vi "ma_Spectrum Averaging (complex) no State.vi"(6 "state info":T2 {"real spectrum" format="%0.2f"; "averages completed" format="%0.2f"; "df" format="%0.2f"; "complex spectrum" format="%0.2f"; "spectrum parameters"."window" items=["Rectangle"=0, "Hanning"=1, "Hamming"=2, "Blackman-Harris"=3, "Exact Blackman"=4, "Blackman"=5, "Flat Top"=6, "4 Term B-Harris "=7, "7 Term B-Harris"=8, "Low Sidelobe"=9, "Blackman Nuttall"=11, "Triangle"=30, "Bartlett-Hanning"=31, "Bohman"=32, "Parzen"=33, "Welch"=34, "Kaiser"=60, "Dolph-Chebyshev"=61, "Gaussian"=62]; "dt" format="%0.2f"; "timestamp" format="%0.2f"; "dt history" format="%0.2f"; "t0 history" format="%0.2f"}, 7 "retrieve last spectrum (F)":bool, 8 "restart averaging (F)":bool, 9 "averaging parameters":T3={"averaging mode"=enum."No averaging", "weighting mode"=enum."Exponential", "number of averages"=10} {"number of averages" min=1}, 10 "df":dbl format="%0.2p", 11 "complex spectrum":cdb[](array[numeric]) format="%0.2p") -> (0 "averages completed":dbl format="%0.2f", 1 "averaging done":bool, 2 "df":dbl format="%0.2p", 3 "averaged complex spectrum":cdb[](array[numeric]) format="%0.2p", 4 "state info":T2 {"real spectrum" format="%0.2f"; "averages completed" format="%0.2f"; "df" format="%0.2f"; "complex spectrum" format="%0.2f"; "spectrum parameters"."window" items=["Rectangle"=0, "Hanning"=1, "Hamming"=2, "Blackman-Harris"=3, "Exact Blackman"=4, "Blackman"=5, "Flat Top"=6, "4 Term B-Harris "=7, "7 Term B-Harris"=8, "Low Sidelobe"=9, "Blackman Nuttall"=11, "Triangle"=30, "Bartlett-Hanning"=31, "Bohman"=32, "Parzen"=33, "Welch"=34, "Kaiser"=60, "Dolph-Chebyshev"=61, "Gaussian"=62]; "dt" format="%0.2f"; "timestamp" format="%0.2f"; "dt history" format="%0.2f"; "t0 history" format="%0.2f"})   [LabVIEW 2020, in "NI_MAPro.lvlib"]
uses:
  NI_MAPro.lvlib
  windowTd.ctl
  NI_AALPro.lvlib
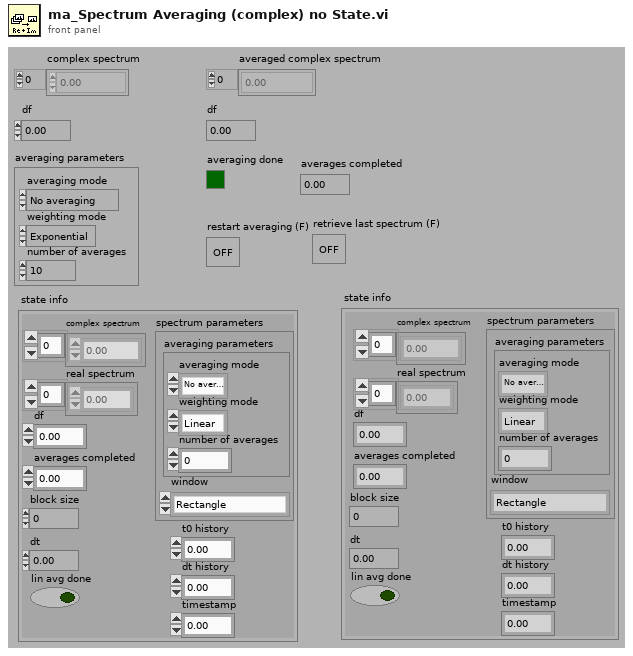
[diagram p1: front panel]
types:
  T1 = typedef "NI_AALPro.lvlib/windowTd.ctl" = u32
  T2 = cluster{"block size":i32, "dt":dbl, "spectrum parameters":cluster{"averaging parameters":cluster{"averaging mode":enum16{"No averaging", "Vector averaging", "RMS averaging", "Peak hold"}, "weighting mode":enum16{"Linear", "Exponential"}, "number of averages":u32}, "window":T1}, "df":dbl, "averages completed":dbl, "complex spectrum":cdb[], "real spectrum":dbl[], "t0 history":dbl, "dt history":dbl, "timestamp":dbl, "lin avg done":bool}
  T3 = cluster{"averaging mode":enum16{"No averaging", "Vector averaging", "RMS averaging", "Peak hold"}, "weighting mode":enum16{"Linear", "Exponential"}, "number of averages":u32}
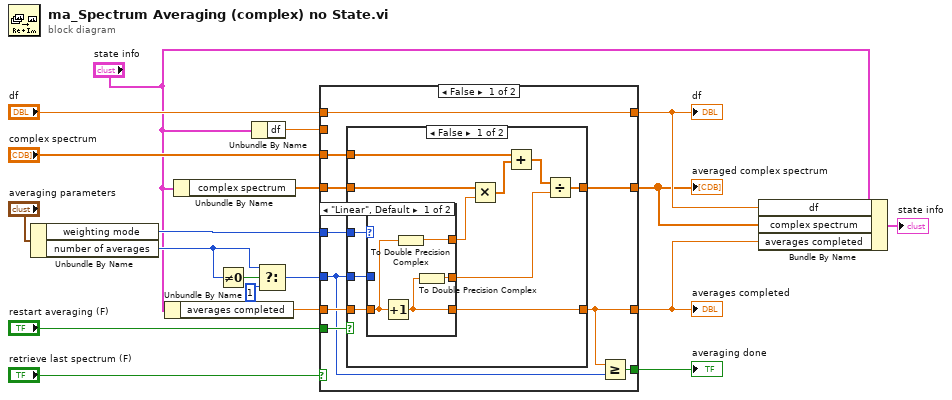
[diagram p0: block diagram]
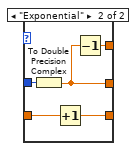
[diagram p2: hidden frame]
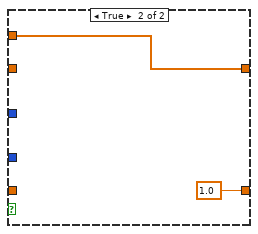
[diagram p3: hidden frame]
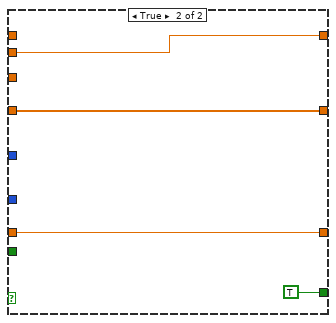
[diagram p4: hidden frame]
diagram:
  n1 = Unbundle By Name("averaging parameters") -> ("weighting mode"=w16:enum16{"Linear", "Exponential"}, "number of averages"=w11:u32)
  n2 = Unbundle By Name("state info") -> ("averages completed"=w6:dbl)
  n3 = Unbundle By Name("state info") -> ("complex spectrum"=w8:cdb[])
  n4 = Not Equal To 0?(x=w11) -> (x != 0?=w12:bool)
  n5 = Unbundle By Name("state info") -> ("df"=w7:dbl)
  n6 = Select(t=w11, s=w12, f=u32 1) -> (s? t:f=w9:u32)
  n7 = case shown="False" "retrieve last spectrum (F)" {
    tunnel: [w29 w55] -> w3
    tunnel: w6 -> [w28 w54]
    tunnel: w8 -> [w27 w55]
    tunnel: w16 -> [w26 _]
    tunnel: "complex spectrum" -> [w25 _]
    tunnel: "restart averaging (F)" -> [w24 _]
    tunnel: w9 -> [w23 _]
    tunnel: [w22 w54] -> w2
    tunnel: [w21 TRUE] -> w15
    tunnel: "df" -> [w20 _]
    tunnel: [w20 w52] -> w4
    tunnel: w7 -> [_ w52]
    frame False {
      n8 = case shown="False" w24 {
        tunnel: [w37 w50] -> w29
        tunnel: [w32 1.0] -> w22
        tunnel: w28 -> [w35 _]
        tunnel: w27 -> [w40 _]
        tunnel: w25 -> [w36 w50]
        tunnel: w26 -> [w33 _]
        tunnel: w23 -> [w30 _]
        frame False {
          n9 = case shown="\"Linear\", Default" w33 {
            tunnel: w35 -> [w43 w48]
            tunnel: [w41 w49] -> w32
            tunnel: [w44 w45] -> w34
            tunnel: [w42 w46] -> w31
            tunnel: w30 -> [_ w47]
            frame "Linear", Default {
              n10 = Increment(x=w43) -> (x+1=w41:dbl)
              n11 = To Double Precision Complex(1:w43) -> (0:w44:cdb)
              n12 = To Double Precision Complex(1:w41) -> (0:w42:cdb)
            }
            frame "Exponential" {
              n13 = To Double Precision Complex(1:w47) -> (0:w46:cdb)
              n14 = Increment(x=w48) -> (x+1=w49:dbl)
              n15 = Decrement(x=w46) -> (x-1=w45:cdb)
            }
          }
          n16 = Multiply(x=w40, y=w34) -> (x*y=w39:cdb[])
          n17 = Add(x=w36, y=w39) -> (x+y=w38:cdb[])
          n18 = Divide(x=w38, y=w31) -> (x/y=w37:cdb[])
        }
        frame True {
        }
      }
      n19 = Greater Or Equal?(x=w22, y=w23) -> (x >= y?=w21:bool)
    }
    frame True {
    }
  }
  "averaged complex spectrum" <- w3
  "averages completed" <- w2
  "averaging done" <- w15
  "df" <- w4
  n20 = Bundle By Name(cluster="state info", "df"=w4, "complex spectrum"=w3, "averages completed"=w2) -> (→"state info":T2)
